vi "Read Result.vi"(8 "error in (no error)":errorcluster, 11 "Result Reply Msg in":refnum<class "Result Reply Msg.lvclass">) -> (0 "error out":errorcluster, 2 "Acquired Result.lvclass":refnum<class "Acquired Result.lvclass">, 3 "Result Reply Msg out":refnum<class "Result Reply Msg.lvclass">)   [LabVIEW 2016, in "Result Reply Msg.lvclass"]
uses:
  Result Reply Msg.lvclass
  NHMFL_Core/Libraries/Instruments/Results/Acquired Result/Acquired Result.lvclass
  Result Reply Msg.lvclass/Result Reply Msg.ctl
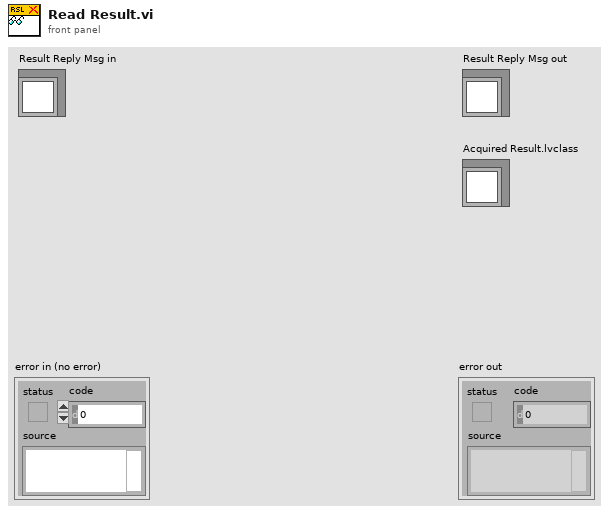
[diagram p1: front panel]
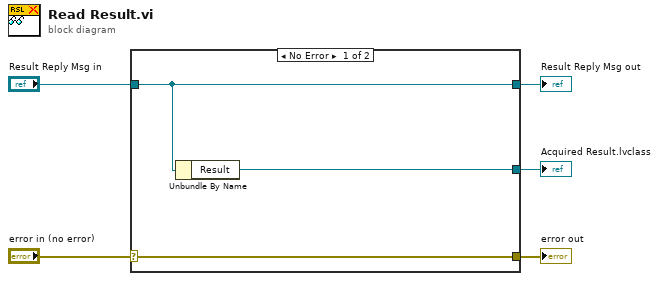
[diagram p0: block diagram]
diagram:
  n1 = case shown="No Error" "error in (no error)" {
    selector: "error in (no error)" -> [w8 w9]
    tunnel: [w8 w9] -> w4
    tunnel: [w7 w10] -> w2
    tunnel: "Result Reply Msg in" -> [w7 w10]
    tunnel: [w6 _] -> w1
    frame No Error {
      n2 = Unbundle By Name(w7) -> ("Result"=w6:refnum<class "Acquired Result.lvclass">)
    }
    frame Error {
    }
  }
  "error out" <- w4
  "Result Reply Msg out" <- w2
  "Acquired Result.lvclass" <- w1
